vi "Convert Data String to Display.vi"(7 "precision (3)":i16=3, 8 "error in (no error)":errorcluster, 9 "endianness (little-endian)":T1(ring), 10 "string data type":T2, 11 "data string":string) -> (0 "error out":errorcluster, 3 "display string":string)   [LabVIEW 2017, in "DSF Core.lvlib"]
uses:
  DSF Core.lvlib
  Typedefs/DSF Data Type.ctl
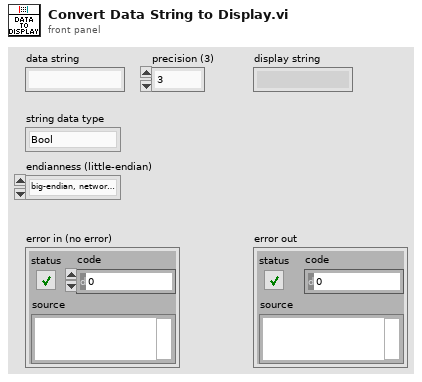
[diagram p1: front panel]
types:
  T1 = enum16{"big-endian, network order", "native, host order", "little-endian"}
  T2 = typedef "DSF Core.lvlib/DSF Data Type.ctl" = enum8{"Bool", "SGL", "DBL", "I8", "I16", "I32", "I64", "U8", "U16", "U32", "U64"}
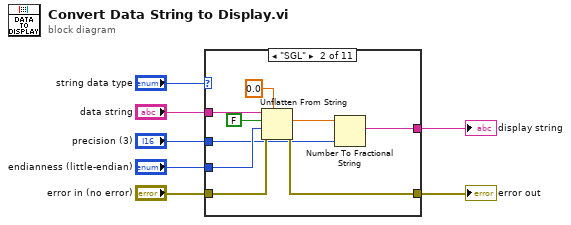
[diagram p0: block diagram]
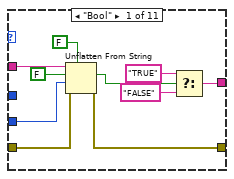
[diagram p2: hidden frame]
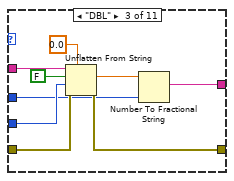
[diagram p3: hidden frame]
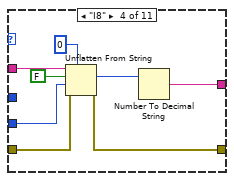
[diagram p4: hidden frame]
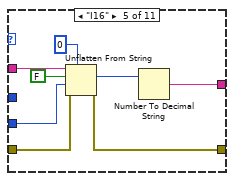
[diagram p5: hidden frame]
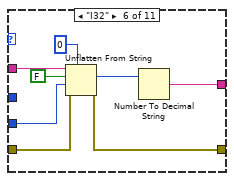
[diagram p6: hidden frame]
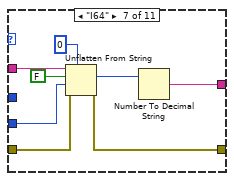
[diagram p7: hidden frame]
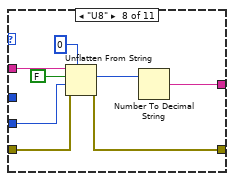
[diagram p8: hidden frame]
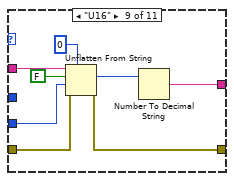
[diagram p9: hidden frame]
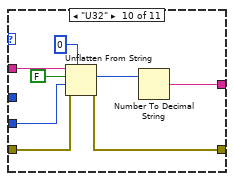
[diagram p10: hidden frame]
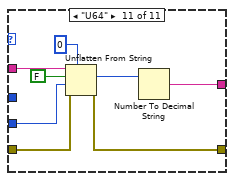
[diagram p11: hidden frame]
diagram:
  n1 = case shown="\"SGL\"" "string data type" {
    tunnel: "error in (no error)" -> [w17 w26 w35 w43 w51 w59 w67 w75 w83 w91 w99]
    tunnel: [w16 w25 w34 w42 w50 w58 w66 w74 w82 w90 w98] -> w4
    tunnel: "endianness (little-endian)" -> [w11 w22 w31 w39 w47 w55 w63 w71 w79 w87 w95]
    tunnel: [w10 w20 w29 w37 w45 w52 w61 w69 w77 w85 w93] -> w7
    tunnel: "data string" -> [w8 w19 w28 w36 w44 w53 w60 w68 w76 w84 w92]
    tunnel: "precision (3)" -> [_ w18 w27 _ _ _ _ _ _ _ _]
    frame "Bool" {
      n2 = Unflatten From String(type=FALSE, binary string=w8, data includes array or string size? (T)=FALSE, byte order (0:big-endian, network order)=w11, error in (no error)=w17) -> (value=w9:bool, error out=w16:errorcluster)  [unwired: 1 out]
      n3 = Select(t="TRUE", s=w9, f="FALSE") -> (s? t:f=w10:string)
    }
    frame "SGL" {
      n4 = Unflatten From String(type=sgl 0.0, binary string=w19, data includes array or string size? (T)=FALSE, byte order (0:big-endian, network order)=w22, error in (no error)=w26) -> (value=w21:sgl, error out=w25:errorcluster)  [unwired: 1 out]
      n5 = Number To Fractional String(number=w21, precision (6)=w18) -> (F-format string=w20:string)  [unwired: 2 in]
    }
    frame "DBL" {
      n6 = Unflatten From String(type=0.0, binary string=w28, data includes array or string size? (T)=FALSE, byte order (0:big-endian, network order)=w31, error in (no error)=w35) -> (value=w30:dbl, error out=w34:errorcluster)  [unwired: 1 out]
      n7 = Number To Fractional String(number=w30, precision (6)=w27) -> (F-format string=w29:string)  [unwired: 2 in]
    }
    frame "I8" {
      n8 = Unflatten From String(type=i8 0, binary string=w36, data includes array or string size? (T)=FALSE, byte order (0:big-endian, network order)=w39, error in (no error)=w43) -> (value=w38:i8, error out=w42:errorcluster)  [unwired: 1 out]
      n9 = Number To Decimal String(number=w38) -> (decimal integer string=w37:string)  [unwired: 1 in]
    }
    frame "I16" {
      n10 = Unflatten From String(type=i16 0, binary string=w44, data includes array or string size? (T)=FALSE, byte order (0:big-endian, network order)=w47, error in (no error)=w51) -> (value=w46:i16, error out=w50:errorcluster)  [unwired: 1 out]
      n11 = Number To Decimal String(number=w46) -> (decimal integer string=w45:string)  [unwired: 1 in]
    }
    frame "I32" {
      n12 = Unflatten From String(type=0, binary string=w53, data includes array or string size? (T)=FALSE, byte order (0:big-endian, network order)=w55, error in (no error)=w59) -> (value=w54:i32, error out=w58:errorcluster)  [unwired: 1 out]
      n13 = Number To Decimal String(number=w54) -> (decimal integer string=w52:string)  [unwired: 1 in]
    }
    frame "I64" {
      n14 = Unflatten From String(type=i64 0, binary string=w60, data includes array or string size? (T)=FALSE, byte order (0:big-endian, network order)=w63, error in (no error)=w67) -> (value=w62:i64, error out=w66:errorcluster)  [unwired: 1 out]
      n15 = Number To Decimal String(number=w62) -> (decimal integer string=w61:string)  [unwired: 1 in]
    }
    frame "U8" {
      n16 = Unflatten From String(type=u8 0, binary string=w68, data includes array or string size? (T)=FALSE, byte order (0:big-endian, network order)=w71, error in (no error)=w75) -> (value=w70:u8, error out=w74:errorcluster)  [unwired: 1 out]
      n17 = Number To Decimal String(number=w70) -> (decimal integer string=w69:string)  [unwired: 1 in]
    }
    frame "U16" {
      n18 = Unflatten From String(type=u16 0, binary string=w76, data includes array or string size? (T)=FALSE, byte order (0:big-endian, network order)=w79, error in (no error)=w83) -> (value=w78:u16, error out=w82:errorcluster)  [unwired: 1 out]
      n19 = Number To Decimal String(number=w78) -> (decimal integer string=w77:string)  [unwired: 1 in]
    }
    frame "U32" {
      n20 = Unflatten From String(type=u32 0, binary string=w84, data includes array or string size? (T)=FALSE, byte order (0:big-endian, network order)=w87, error in (no error)=w91) -> (value=w86:u32, error out=w90:errorcluster)  [unwired: 1 out]
      n21 = Number To Decimal String(number=w86) -> (decimal integer string=w85:string)  [unwired: 1 in]
    }
    frame "U64" {
      n22 = Unflatten From String(type=u64 0, binary string=w92, data includes array or string size? (T)=FALSE, byte order (0:big-endian, network order)=w95, error in (no error)=w99) -> (value=w94:u64, error out=w98:errorcluster)  [unwired: 1 out]
      n23 = Number To Decimal String(number=w94) -> (decimal integer string=w93:string)  [unwired: 1 in]
    }
  }
  "display string" <- w7
  "error out" <- w4
